vi "Draw Field.vi"(8 "error in (no error)":errorcluster, 10 "Field Size":T1, 11 "Field Drawer in":refnum<class "Field Drawer.lvclass">) -> (0 "error out":errorcluster, 3 "Field Drawer out":refnum<class "Field Drawer.lvclass">)   [LabVIEW 2022 SP3, in "Vision.lvlib" / "Field Drawer.lvlib" / "Field Drawer.lvclass"]
uses:
  Field Drawer.lvclass
  Old vision/Controls/Field Size.ctl
  <vilib>/Utility/miscctls.llb/LVBoundsTypeDef.ctl
  Project.ctl
  Field Drawer.lvclass/Field Drawer.ctl
panel:
  in  "rect":T2
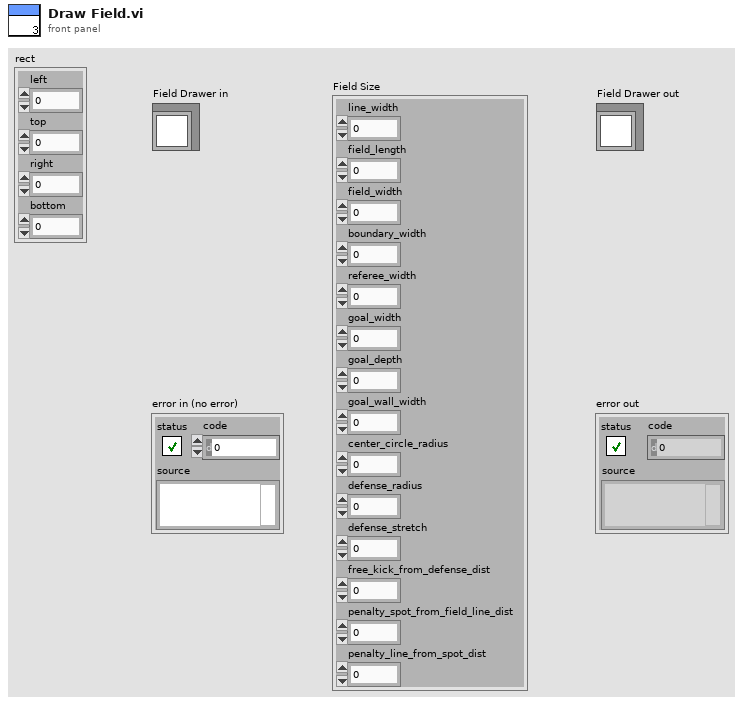
[diagram p1: front panel]
types:
  T1 = typedef "Field Size.ctl" = cluster{"line_width":u32, "field_length":u32, "field_width":u32, "boundary_width":u32, "referee_width":u32, "goal_width":u32, "goal_depth":u32, "goal_wall_width":u32, "center_circle_radius":u32, "defense_radius":u32, "defense_stretch":u32, "free_kick_from_defense_dist":u32, "penalty_spot_from_field_line_dist":u32, "penalty_line_from_spot_dist":u32}
  T2 = cluster{"left":i16, "top":i16, "right":i16, "bottom":i16}
  T3 = typedef "Project.ctl" = enum16{"SSL", "VSS"}
  T4 = typedef "LVBoundsTypeDef.ctl" = cluster{"Width":u32, "Height":u32}
  T5 = cluster{"Width":i16, "Style":enum32{"Solid", "Dash", "Dot", "DashDot", "DashDotDot"}}
  T6 = cluster{"line_width":dbl, "field_length":dbl, "field_width":dbl, "boundary_width":dbl, "referee_width":dbl, "goal_width":dbl, "goal_depth":dbl, "goal_wall_width":dbl, "center_circle_radius":dbl, "defense_radius":dbl, "defense_stretch":dbl, "free_kick_from_defense_dist":dbl, "penalty_spot_from_field_line_dist":dbl, "penalty_line_from_spot_dist":dbl}
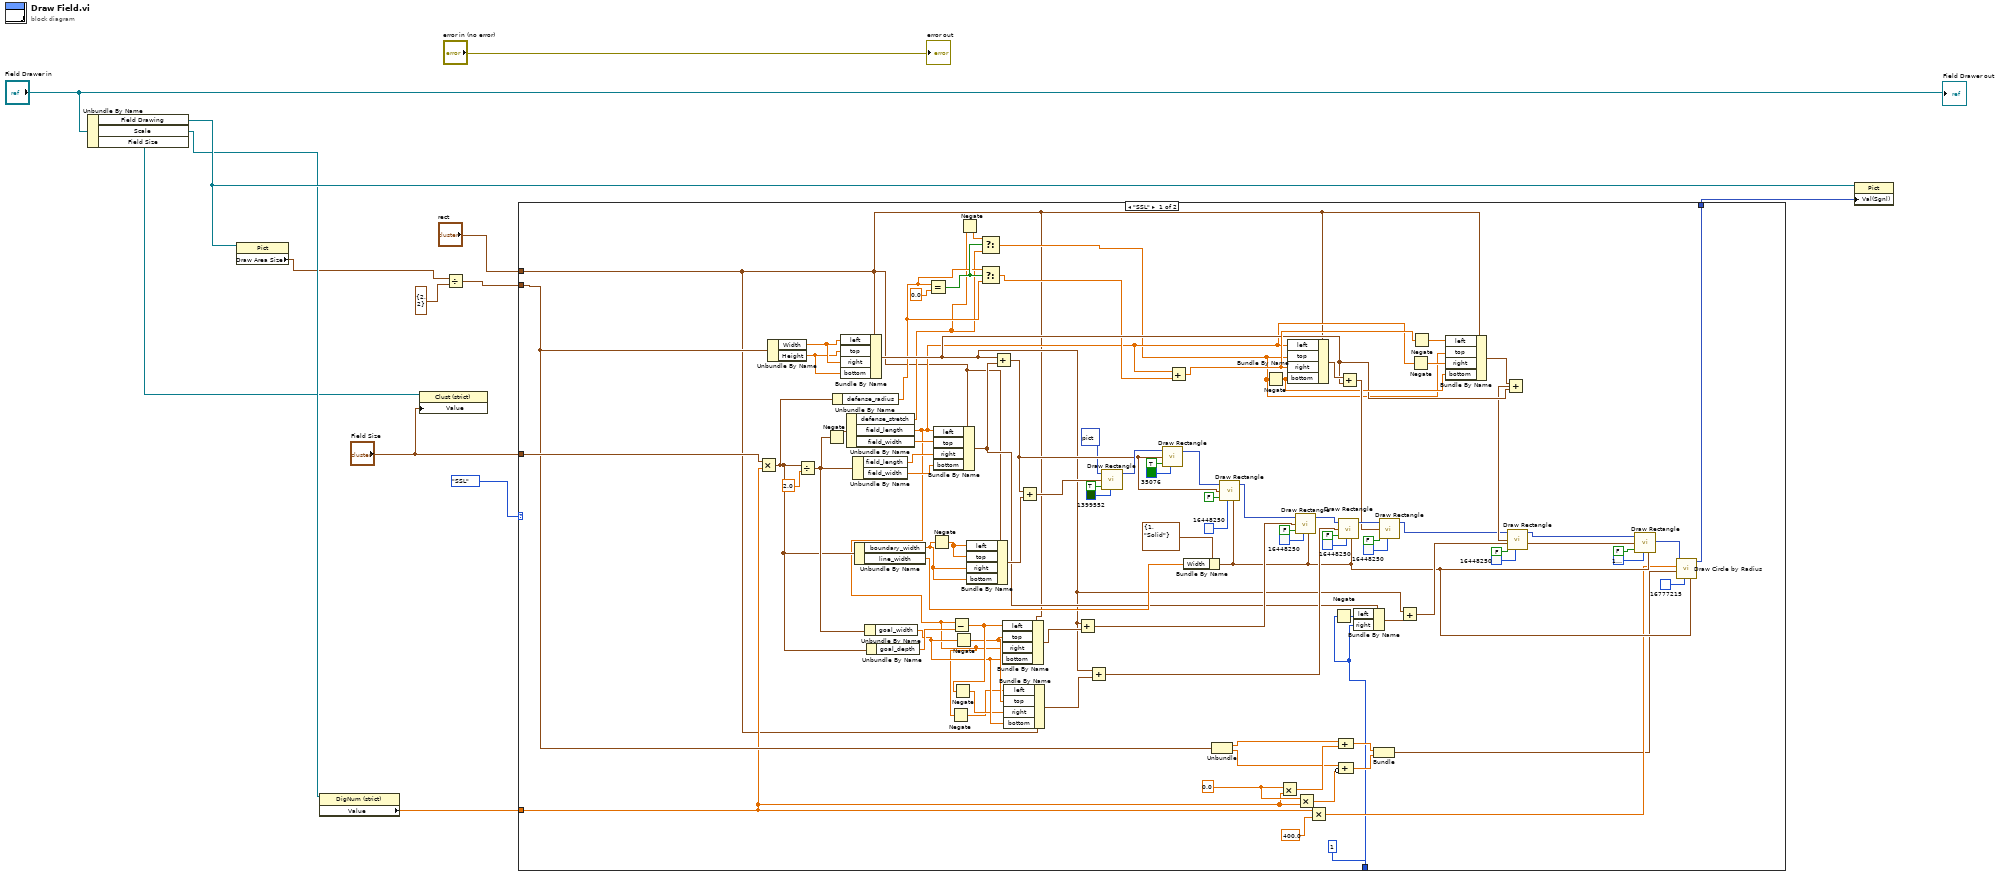
[diagram p0: block diagram]
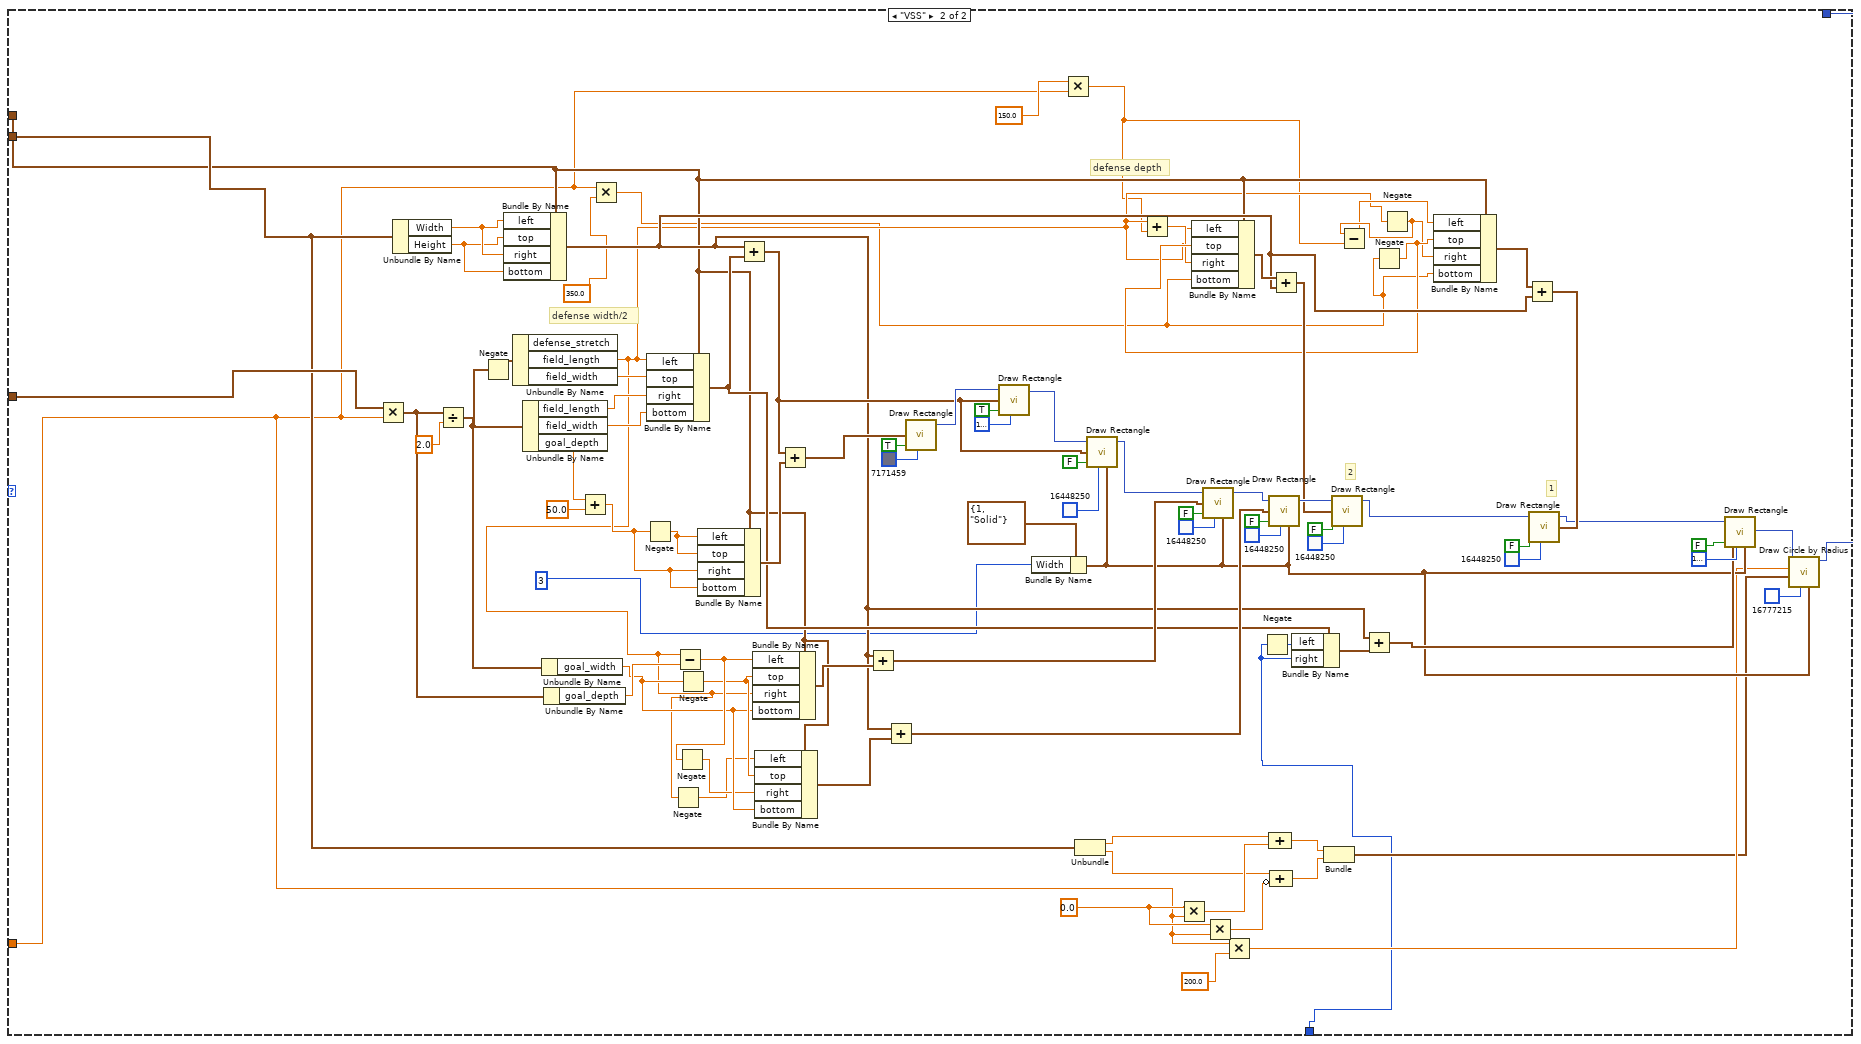
[diagram p2: hidden frame]
diagram:
  n1 = Unbundle By Name("Field Drawer in") -> ("Field Drawing"=w12:refnum<vi>, "Scale"=w11:refnum<vi>, "Field Size"=w3:refnum<vi>)
  n2 = property class="Pict"(reference=w12) -> ("Draw Area Size"=w1:T4)  [unwired: 1 in, 2 out]
  n3 = property class="DigNum (strict)"(reference=w11) -> ("Value"=w10:dbl)  [unwired: 1 in, 2 out]
  n4 = property class="Clust (strict)"(reference=w3, "Value"="Field Size") -> ()  [unwired: 1 in, 2 out]
  n5 = Divide(x=w1, y=T4 {"Width"=2, "Height"=2}) -> (x/y=w9:cluster{"Width":dbl, "Height":dbl})
  n6 = case shown="\"SSL\"" Project."SSL" ("Project") {
    tunnel: "Field Size" -> [w21 w123]
    tunnel: w9 -> [w20 w122]
    tunnel: w10 -> [w19 w107]
    tunnel: "rect" -> [w18 w121]
    tunnel: i16 1 ("left") -> [w17 w120]
    tunnel: [w16 w119] -> w4
    frame "SSL" {
      w47 = 0.0 ("x")
      n7 = Multiply(x=w21, y=w19) -> (x*y=w46:T6)
      n8 = Unbundle By Name(w20) -> ("Width"=w101:dbl, "Height"=w100:dbl)
      n9 = Divide(x=w46, y=2.0) -> (x/y=w77:T6)
      n10 = Negate(x=w77) -> (-x=w96:T6)
      n11 = Unbundle By Name(w46) -> ("defense_radius"=w23:dbl)
      n12 = Bundle By Name(cluster=w18, "left"=w101, "top"=w100, "right"=w101, "bottom"=w100) -> (w33:T2)
      n13 = Unbundle By Name(w96) -> ("defense_stretch"=w22:dbl, "field_length"=w28:dbl, "field_width"=w99:dbl)
      n14 = Unbundle By Name(w77) -> ("field_length"=w98:dbl, "field_width"=w97:dbl)
      n15 = Unbundle By Name(w46) -> ("boundary_width"=w94:dbl, "line_width"=w84:dbl)
      n16 = Unbundle By Name(w77) -> ("goal_width"=w71:dbl)
      n17 = Unbundle By Name(w46) -> ("goal_depth"=w76:dbl)
      n18 = Equal?(x=w23, y=0.0) -> (x = y?=w30:bool)
      n19 = Negate(x=w94) -> (-x=w95:dbl)
      n20 = Bundle By Name(cluster=w18, "left"=w28, "top"=w99, "right"=w98, "bottom"=w97) -> (w64:T2)
      n21 = Negate(x=w28) -> (-x=w67:dbl)
      n22 = Subtract(x=w28, y=w76) -> (x-y=w73:dbl)
      n23 = Negate(x=w73) -> (-x=w68:dbl)
      n24 = Negate(x=w71) -> (-x=w72:dbl)
      n25 = Negate(x=w22) -> (-x=w26:dbl)
      n26 = Bundle By Name(cluster=w18, "left"=w95, "top"=w95, "right"=w94, "bottom"=w94) -> (w93:T2)
      n27 = Select(t=w26, s=w30, f=w22) -> (s? t:f=w27:dbl)
      n28 = Select(t=w23, s=w30, f=w23) -> (s? t:f=w29:dbl)
      n29 = Add(x=w33, y=w64) -> (x+y=w57:T2)
      n30 = Bundle By Name(cluster=w18, "left"=w73, "top"=w72, "right"=w28, "bottom"=w71) -> (w75:T2)
      n31 = Bundle By Name(cluster=w18, "left"=w67, "top"=w72, "right"=w68, "bottom"=w71) -> (w70:T2)
      n32 = Add(x=w57, y=w93) -> (x+y=w90:T2)
      n33 = Add(x=w33, y=w75) -> (x+y=w74:T2)
      n34 = Add(x=w33, y=w70) -> (x+y=w69:T2)
      n35 = call <vilib>:"Draw Rectangle.vi"("picture"=picture data[5B], "rect"=w90, "fill?(F)"=TRUE, "color(black)"=u32 1399552) -> ("new picture"=w89:picture)  [unwired: 5 in]
      n36 = call <vilib>:"Draw Rectangle.vi"("picture"=w89, "rect"=w57, "fill?(F)"=TRUE, "color(black)"=u32 35076) -> ("new picture"=w86:picture)  [unwired: 5 in]
      n37 = Add(x=w28, y=w29) -> (x+y=w39:dbl)
      n38 = Bundle By Name(cluster=T5 {"Width"=1, "Style"=enum."Solid"} ("pen"), "Width"=w84) -> (w58:T5)
      n39 = Unbundle(w20) -> ("Width"=w55:dbl, "Height"=w52:dbl)
      n40 = call <vilib>:"Draw Rectangle.vi"("picture"=w86, "rect"=w57, "fill?(F)"=FALSE, "color(black)"=u32 16448250, "pen"=w58) -> ("new picture"=w81:picture)  [unwired: 4 in]
      n41 = Negate(x=w27) -> (-x=w37:dbl)
      n42 = Multiply(x=w47, y=w19) -> (x*y=w54:dbl)
      n43 = Bundle By Name(cluster=w18, "left"=w28, "top"=w27, "right"=w39, "bottom"=w37) -> (w42:T2)
      n44 = call <vilib>:"Draw Rectangle.vi"("picture"=w81, "rect"=w74, "fill?(F)"=FALSE, "color(black)"=u32 16448250, "pen"=w58) -> ("new picture"=w78:picture)  [unwired: 4 in]
      n45 = Multiply(x=w47, y=w19) -> (x*y=w51:dbl)
      n46 = Multiply(x=w19, y=sgl 400.0 ("radius")) -> (x*y=w49:dbl)
      n47 = Negate(x=w17) -> (-x=w61:i16)
      n48 = call <vilib>:"Draw Rectangle.vi"("picture"=w78, "rect"=w69, "fill?(F)"=FALSE, "color(black)"=u32 16448250, "pen"=w58) -> ("new picture"=w43:picture)  [unwired: 4 in]
      n49 = Compound Arithmetic op=ADD(w55, w54) -> (w53:dbl)
      n50 = Compound Arithmetic op=ADD(w52, invert w51) -> (w50:dbl)
      n51 = Add(x=w42, y=w33) -> (x+y=w41:T2)
      n52 = Bundle By Name(cluster=w64, "left"=w61, "right"=w17) -> (w63:T2)
      n53 = Bundle(w53, w50) -> (w48:cluster{dbl, dbl})  [unwired: 1 in]
      n54 = call <vilib>:"Draw Rectangle.vi"("picture"=w43, "rect"=w41, "fill?(F)"=FALSE, "color(black)"=u32 16448250) -> ("new picture"=w25:picture)  [unwired: 5 in]
      n55 = Add(x=w33, y=w63) -> (x+y=w62:T2)
      n56 = Negate(x=w28) -> (-x=w40:dbl)
      n57 = Negate(x=w39) -> (-x=w38:dbl)
      n58 = Bundle By Name(cluster=w18, "left"=w38, "top"=w27, "right"=w40, "bottom"=w37) -> (w34:T2)
      n59 = Add(x=w34, y=w33) -> (x+y=w32:T2)
      n60 = call <vilib>:"Draw Rectangle.vi"("picture"=w25, "rect"=w32, "fill?(F)"=FALSE, "color(black)"=u32 16448250) -> ("new picture"=w24:picture)  [unwired: 5 in]
      n61 = call <vilib>:"Draw Rectangle.vi"("picture"=w24, "rect"=w62, "fill?(F)"=FALSE, "color(black)"=u32 16777226, "pen"=w58) -> ("new picture"=w60:picture)  [unwired: 4 in]
      n62 = call <vilib>:"Draw Circle by Radius.vi"("pen"=w58, "color(black)"=u32 16777215, "pixel center"=w48, "radius"=w49, "picture"=w60) -> ("new picture"=w16:picture)  [unwired: 6 in]
    }
    frame "VSS" {
      w137 = 0.0 ("x")
      # "defense width/2"
      # "defense depth"
      # "1"
      # "2"
      n63 = Multiply(x=w123, y=w107) -> (x*y=w136:T6)
      n64 = Unbundle By Name(w122) -> ("Width"=w189:dbl, "Height"=w188:dbl)
      n65 = Divide(x=w136, y=2.0) -> (x/y=w167:T6)
      n66 = Negate(x=w167) -> (-x=w184:T6)
      n67 = Bundle By Name(cluster=w121, "left"=w189, "top"=w188, "right"=w189, "bottom"=w188) -> (w127:T2)
      n68 = Unbundle By Name(w184) -> ("field_length"=w110:dbl, "field_width"=w187:dbl)  [unwired: 1 out]
      n69 = Unbundle By Name(w167) -> ("field_length"=w186:dbl, "field_width"=w185:dbl, "goal_depth"=w117:dbl)
      n70 = Unbundle By Name(w167) -> ("goal_width"=w161:dbl)
      n71 = Unbundle By Name(w136) -> ("goal_depth"=w166:dbl)
      n72 = Add(x=w117, y=50.0) -> (x+y=w116:dbl)
      n73 = Multiply(x=w107, y=350.0) -> (x*y=w106:dbl)
      n74 = Negate(x=w116) -> (-x=w183:dbl)
      n75 = Bundle By Name(cluster=w121, "left"=w110, "top"=w187, "right"=w186, "bottom"=w185) -> (w154:T2)
      n76 = Negate(x=w110) -> (-x=w157:dbl)
      n77 = Subtract(x=w110, y=w166) -> (x-y=w163:dbl)
      n78 = Negate(x=w163) -> (-x=w158:dbl)
      n79 = Negate(x=w161) -> (-x=w162:dbl)
      n80 = Bundle By Name(cluster=w121, "left"=w183, "top"=w183, "right"=w116, "bottom"=w116) -> (w182:T2)
      n81 = Add(x=w127, y=w154) -> (x+y=w147:T2)
      n82 = Bundle By Name(cluster=w121, "left"=w163, "top"=w162, "right"=w110, "bottom"=w161) -> (w165:T2)
      n83 = Bundle By Name(cluster=w121, "left"=w157, "top"=w162, "right"=w158, "bottom"=w161) -> (w160:T2)
      n84 = Add(x=w147, y=w182) -> (x+y=w179:T2)
      n85 = Add(x=w127, y=w165) -> (x+y=w164:T2)
      n86 = Add(x=w127, y=w160) -> (x+y=w159:T2)
      n87 = call <vilib>:"Draw Rectangle.vi"("rect"=w179, "fill?(F)"=TRUE, "color(black)"=u32 7171459) -> ("new picture"=w178:picture)  [unwired: 6 in]
      n88 = call <vilib>:"Draw Rectangle.vi"("picture"=w178, "rect"=w147, "fill?(F)"=TRUE, "color(black)"=u32 16777222) -> ("new picture"=w175:picture)  [unwired: 5 in]
      n89 = Bundle By Name(cluster=T5 {"Width"=1, "Style"=enum."Solid"} ("pen"), "Width"=i16 3) -> (w148:T5)
      n90 = Multiply(x=150.0, y=w107) -> (x*y=w105:dbl)
      n91 = Unbundle(w122) -> ("Width"=w145:dbl, "Height"=w142:dbl)
      n92 = call <vilib>:"Draw Rectangle.vi"("picture"=w175, "rect"=w147, "fill?(F)"=FALSE, "color(black)"=u32 16448250, "pen"=w148) -> ("new picture"=w171:picture)  [unwired: 4 in]
      n93 = Add(x=w110, y=w105) -> (x+y=w111:dbl)
      n94 = Multiply(x=w137, y=w107) -> (x*y=w144:dbl)
      n95 = call <vilib>:"Draw Rectangle.vi"("picture"=w171, "rect"=w164, "fill?(F)"=FALSE, "color(black)"=u32 16448250, "pen"=w148) -> ("new picture"=w168:picture)  [unwired: 4 in]
      n96 = Multiply(x=w137, y=w107) -> (x*y=w141:dbl)
      n97 = Multiply(x=w107, y=sgl 200.0 ("radius")) -> (x*y=w139:dbl)
      n98 = Negate(x=w120) -> (-x=w151:i16)
      n99 = call <vilib>:"Draw Rectangle.vi"("picture"=w168, "rect"=w159, "fill?(F)"=FALSE, "color(black)"=u32 16448250, "pen"=w148) -> ("new picture"=w133:picture)  [unwired: 4 in]
      n100 = Compound Arithmetic op=ADD(w145, w144) -> (w143:dbl)
      n101 = Compound Arithmetic op=ADD(w142, invert w141) -> (w140:dbl)
      n102 = Bundle By Name(cluster=w154, "left"=w151, "right"=w120) -> (w153:T2)
      n103 = Bundle(w143, w140) -> (w138:cluster{dbl, dbl})  [unwired: 1 in]
      n104 = Add(x=w127, y=w153) -> (x+y=w152:T2)
      n105 = Negate(x=w106) -> (-x=w114:dbl)
      n106 = Bundle By Name(cluster=w121, "left"=w110, "top"=w114, "right"=w111, "bottom"=w106) -> (w132:T2)
      n107 = Add(x=w132, y=w127) -> (x+y=w131:T2)
      n108 = call <vilib>:"Draw Rectangle.vi"("picture"=w133, "rect"=w131, "fill?(F)"=FALSE, "color(black)"=u32 16448250) -> ("new picture"=w125:picture)  [unwired: 5 in]
      n109 = Negate(x=w110) -> (-x=w113:dbl)
      n110 = Subtract(x=w113, y=w105) -> (x-y=w112:dbl)
      n111 = Bundle By Name(cluster=w121, "left"=w112, "top"=w114, "right"=w113, "bottom"=w106) -> (w128:T2)
      n112 = Add(x=w128, y=w127) -> (x+y=w126:T2)
      n113 = call <vilib>:"Draw Rectangle.vi"("picture"=w125, "rect"=w126, "fill?(F)"=FALSE, "color(black)"=u32 16448250) -> ("new picture"=w124:picture)  [unwired: 5 in]
      n114 = call <vilib>:"Draw Rectangle.vi"("picture"=w124, "rect"=w152, "fill?(F)"=FALSE, "color(black)"=u32 16777226, "pen"=w148) -> ("new picture"=w150:picture)  [unwired: 4 in]
      n115 = call <vilib>:"Draw Circle by Radius.vi"("pen"=w148, "color(black)"=u32 16777215, "pixel center"=w138, "radius"=w139, "picture"=w150) -> ("new picture"=w119:picture)  [unwired: 6 in]
    }
  }
  n116 = property class="Pict"(reference=w12, "Val(Sgnl)"=w4) -> ()  [unwired: 1 in, 2 out]
  "error out" <- "error in (no error)"
  "Field Drawer out" <- "Field Drawer in"
